vi "server_not_working.vi"() -> ()   [LabVIEW 2012]
panel:
  in  "Settings":T1(array[cluster])
  out "server ID":u32
  out "welcome message":string
  in  "Server Name":string="LabVIEW Server"
  in  "manager":T2={"address"="localhost", "port"=7682, "password"=""}
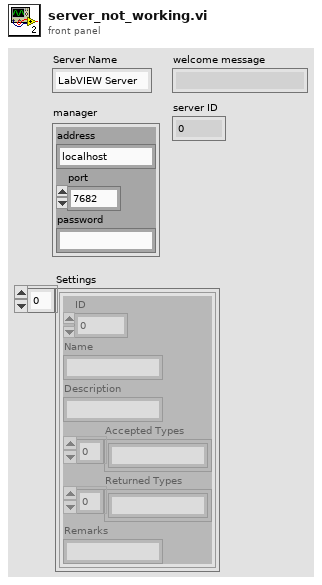
[diagram p1: front panel]
types:
  T1 = cluster{"ID":u32, "Name":string, "Description":string, "Accepted Types":string[], "Returned Types":string[], "Remarks":string}[]
  T2 = cluster{"address":string, "port":u16, "password":string}
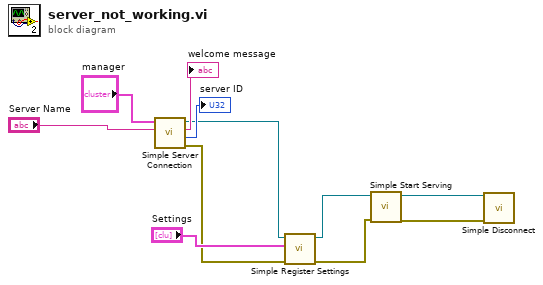
[diagram p0: block diagram]
diagram:
  n1 = call <userlib>:"Simple Server Connection.vi"("connection name (LabVIEW Server)"="Server Name", "manager"="manager") -> ("error out"=w6:errorcluster, "server ID"=→"server ID":u32, "welcome message"=→"welcome message":string, "connection ID out"=w5:refnum<k5>)  [unwired: 2 in]
  n2 = call <userlib>:"Simple Register Settings.vi"("error in (no error)"=w6, "Settings"="Settings", "connection ID"=w5) -> ("error out"=w3:errorcluster, "connection ID out"=w4:refnum<k5>)  [unwired: 3 in]
  n3 = call <userlib>:"Simple Start Serving.vi"("error in (no error)"=w3, "connection ID"=w4) -> ("error out"=w1:errorcluster, "connection ID out"=w2:refnum<k5>)  [unwired: 4 in]
  n4 = call <userlib>:"Simple Disconnect.vi"("error in (no error)"=w1, "connection ID"=w2) -> ()  [unwired: 5 in, 1 out]
